vi "Write Channels and optional channel names.vi"(10 "Channels and optional channel names":cluster{"Enabled":bool, "Channel name":string}[](array[cluster])=[{"Enabled"=TRUE, "Channel name"=""}, {"Enabled"=FALSE, "Channel name"=""}, {"Enabled"=FALSE, "Channel name"=""}, {"Enabled"=FALSE, "Channel name"=""}], 11 "Oscilloscope in":refnum<class "Oscilloscope.lvclass">) -> (3 "Oscilloscope out":refnum<class "Oscilloscope.lvclass">)   [LabVIEW 2020, in "Oscilloscope.lvclass"]
uses:
  Oscilloscope.lvclass
  Oscilloscope.lvclass/Oscilloscope.ctl
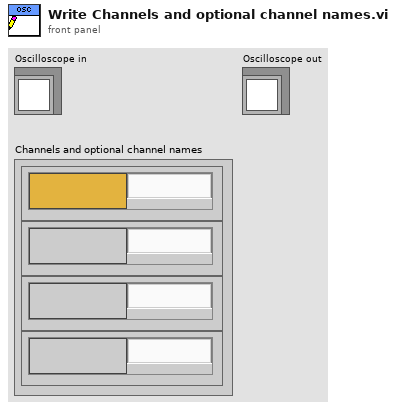
[diagram p1: front panel]
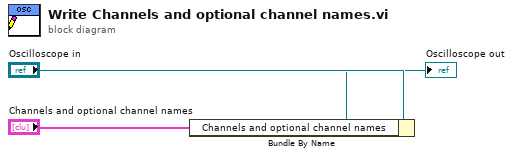
[diagram p0: block diagram]
diagram:
  n1 = Bundle By Name(cluster="Oscilloscope in", "Channels and optional channel names"="Channels and optional channel names") -> (→"Oscilloscope out":refnum<class "Oscilloscope.lvclass">)
